vi "Read port.vi"(9 "Downloader in":refnum<class "Downloader.lvclass">) -> (3 "Downloader out":refnum<class "Downloader.lvclass">, 4 "port":u16=9090)   [LabVIEW 2014, in "Raspberry Pi Compatible Compiler for LabVIEW.lvlib" / "Downloader.lvclass"]
uses:
  Downloader.lvclass
  Downloader.lvclass/Downloader.ctl
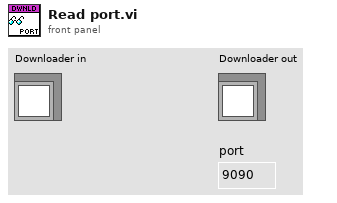
[diagram p1: front panel]
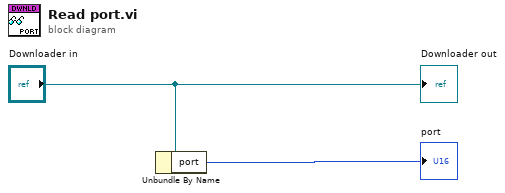
[diagram p0: block diagram]
diagram:
  n1 = Unbundle By Name("Downloader in") -> ("port"=→"port":u16)
  "Downloader out" <- "Downloader in"
